vi "set_libraryWhitelist.vi"(0 "Host_Reference":refnum<class "HGF_Reference.lvclass">, 2 "timeout in ms (-1)":i32=-1, 5 "error in (no error)":errorcluster) -> (14 "dup Host_Reference":refnum<class "HGF_Reference.lvclass">, 19 "error out":errorcluster)   [LabVIEW 2009, in "MoAgSy.lvlib" / "MoAgSy_Host.lvclass"]
doc: "<B>public</B> VI changes referenced hosts library whitelist.\nAgents that belong to a whitelisted library are startet at this host irrespective of the hosts security settings.\n<B>VI frontpanel has to be shown at vi call.</B>\n\nF.Berck@gsi.de\nGSI Darmstadt 2009"
uses:
  MoAgSy_Host.lvclass
  HGF_BaseClasses/HGF_Reference/HGF_Reference.lvclass
panel:
  in  "remove empty":bool
  in  "clear":bool
  in  "Library Whitelist":string[](array[string])
  in  "Cancel":bool
  in  "Apply":bool
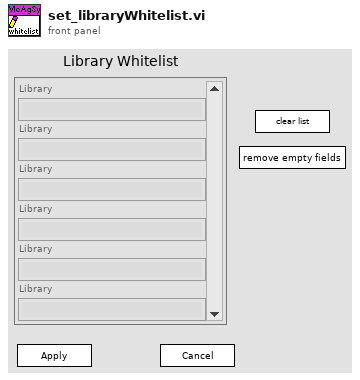
[diagram p1: front panel]
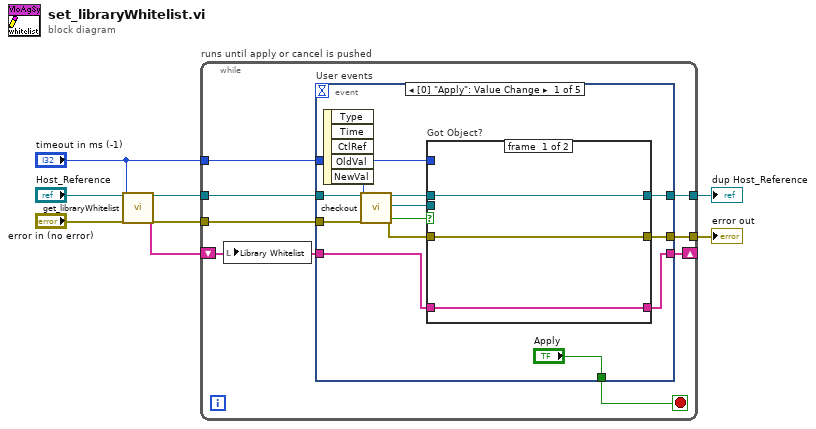
[diagram p0: block diagram]
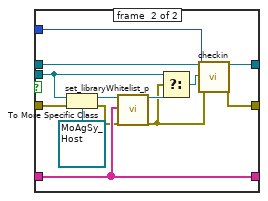
[diagram p2: hidden frame]
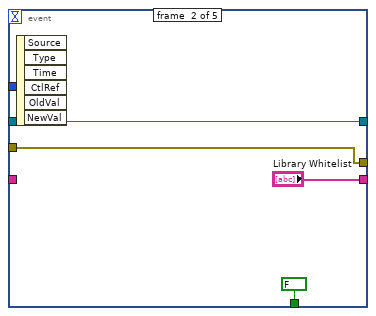
[diagram p3: hidden frame]
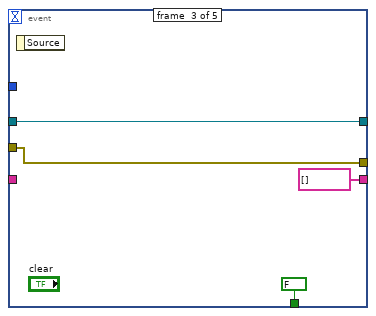
[diagram p4: hidden frame]
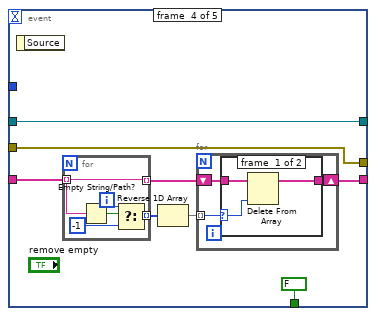
[diagram p5: hidden frame]
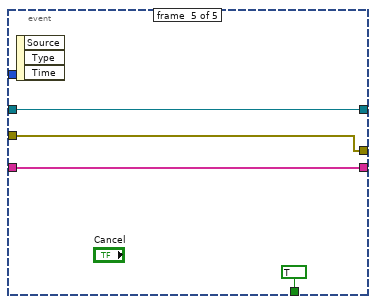
[diagram p7: hidden frame]
diagram:
  n1 = call "get_libraryWhitelist.vi"("Host_Reference"="Host_Reference", "timeout in ms (-1)"="timeout in ms (-1)", "error in (no error)"="error in (no error)") -> ("dup Host_Reference"=w5:refnum<class "HGF_Reference.lvclass">, "Library Whitelist"=w3:string[], "error out"=w4:errorcluster)  [unwired: 14 out]
  n2 = while "runs until apply or cancel is pushed" {
    tunnel: [w16] -> w2
    tunnel: [w15] -> w1
    tunnel: w5 -> [w14]
    tunnel: "timeout in ms (-1)" -> [w13]
    tunnel: w4 -> [w12]
    shift-right: [w10] -> _
    shift-left: w3 -> [w9]
    stop <- w11 stop-if-true
    n3 = local write "Library Whitelist"(w9) -> ()
    n4 = event "User events" shown="[0] \"Apply\": Value Change" {
      selector: _ -> [_ _ _ _ _]
      dyn-events: _ -> [_ _ _ _ _]
      timeout: _ -> [_ _ _ _ _]
      tunnel: [w28 w48 w51 w54 w75] -> w15
      tunnel: [w27 w47 w50 w60 w76] -> w16
      tunnel: w13 -> [w23 _ _ _ _]
      tunnel: w14 -> [w22 w47 w50 w60 w76]
      tunnel: w12 -> [w21 w48 w51 w54 w75]
      tunnel: w9 -> [w18 _ _ w59 w74]
      tunnel: ["Apply" FALSE ("Cancel") FALSE ("Cancel") FALSE ("Cancel") TRUE ("Cancel")] -> w11
      tunnel: [w19 "Library Whitelist" string[] [] ("Library Blacklist") w55 w74] -> w10
      event #0 {
        n5 = event-data() -> ()  [unwired: 6 out]
        n6 = call "checkout.vi"("HGF_Reference"=w22, "timeout in ms (-1)"=w23, "error in (no error)"=w21) -> ("dup HGF_Reference"=w26:refnum<class "HGF_Reference.lvclass">, "Object"=w24:refnum<class>, "got object?"=w25:bool, "error out"=w20:errorcluster)  [unwired: 13 out]
        n7 = case "Got Object?" shown="False" w25 {
          tunnel: w24 -> [_ w38]
          tunnel: w26 -> [w31 w43]
          tunnel: [w31 w42] -> w27
          tunnel: w23 -> [_ w41]
          tunnel: [w30 w40] -> w28
          tunnel: w20 -> [w30 w39]
          tunnel: w18 -> [w29 w33]
          tunnel: [w29 w33] -> w19
          frame #0 {
          }
          frame #1 {
            n8 = To More Specific Class(target class=refnum<class "MoAgSy_Host.lvclass"> refnum ("MoAgSy.lvlib:MoAgSy_Host.lvclass"), reference=w38, error in=w39) -> (specific class reference=w36:refnum<class "MoAgSy_Host.lvclass">, error out=w32:errorcluster)
            n9 = call "set_libraryWhitelist_p.vi"("MoAgSy_Host"=w36, "Library Whitelist"=w33, "error in (no error)"=w32) -> ("dup MoAgSy_Host"=w35:refnum<class "MoAgSy_Host.lvclass">, "error out"=w34:errorcluster)  [unwired: 15 out]
            n10 = Select(t=w38, s=w34, f=w35) -> (s? t:f=w37:refnum<class>)
            n11 = call "checkin.vi"("HGF_Reference"=w43, "Object"=w37, "timeout /ms (-1)"=w41, "error in (no error)"=w34) -> ("dup HGF_Reference"=w42:refnum<class "HGF_Reference.lvclass">, "error out"=w40:errorcluster)  [unwired: 14 out]
          }
        }
      }
      event #1 {
        n12 = event-data() -> ()  [unwired: 7 out]
      }
      event #2 {
        n13 = event-data() -> ()  [unwired: 2 out]
      }
      event #3 {
        n14 = event-data() -> ()  [unwired: 2 out]
        n15 = for {
          tunnel: w59 -> [w68] mode=indexing
          tunnel: [w69] -> w58 mode=indexing
          tunnel: [w68] -> w57 mode=indexing
          i -> [w71]
          n16 = Empty String/Path?(string/path=w68) -> (empty?=w72:bool)
          n17 = Select(t=w71, s=w72, f=-1) -> (s? t:f=w69:i32)
        }
        n18 = Reverse 1D Array(array=w58) -> (reversed array=w56:i32[])
        n19 = for {
          tunnel: w56 -> [w63] mode=indexing
          shift-right: [w61] -> w55
          shift-left: w57 -> [w62]
          n20 = case shown="0, Default" w63 {
            selector: w63 -> [w64 _]
            tunnel: [w65 w67] -> w61
            tunnel: w62 -> [w66 w67]
            frame #0 {
              n21 = Delete From Array(array=w66, index=w64) -> (array with subset deleted=w65:string[])  [unwired: 1 in, 1 out]
            }
            frame #1 {
            }
          }
        }
      }
      event #4 {
        n22 = event-data() -> ()  [unwired: 4 out]
      }
    }
  }
  "dup Host_Reference" <- w2
  "error out" <- w1
